vi "2D_Data_Interp.vi"() -> ()   [LabVIEW 2016]
uses:
  <vilib>/Math Plots/3D Math Plots/3D Surface/3D Surface XCtrl/3D Surface.xctl
  <vilib>/gmath/interp.llb/Interpolate 2D (2d X,Y).vi
  <vilib>/gmath/interp.llb/Create Mesh Grid (2D) (x,y arrays).vi
  <vilib>/Math Plots/3D Math Plots/3D Surface/3D Surface Datatype/Public/Plot Helper (Matrix).vi
  <vilib>/gmath/NI_Gmath.lvlib
  <vilib>/Math Plots/3D Math Plots/3D Surface/3D Surface Datatype/3D Surface Datatype.lvclass
  <vilib>/measure/NI_MABase.lvlib
  <vilib>/picture/3D Picture Control/NI_3D Picture Control.lvlib
panel:
  in  "Differential Conductance":dbl[][](graph)=[[172.002], [172.014], [172.02], [172.032], [172.05], [172.038], [171.99], [171.984], [172.008], [172.02], [172.038], [172.032], [172.008], [171.99], [171.984], [171.99], [172.008], [172.02], [172.032], [171.996], [172.002], [172.014], [172.032], [172.056], [172.056], [172.038], [172.008], [171.996], [172.014], [172.026], [172.032], [172.044], [172.008], [171.996], [171.99], [172.014], [172.032], [172.038], [172.032], [171.99], [171.984], [171.996], [172.014], [172.032], [172.026], [172.002], [171.99], [171.996], [172.02], [172.038], [172.05], [172.032], [172.002], [172.008], [172.014], [172.032], [172.044], [172.056], [172.044], [172.002], [171.996], [172.002], [172.026], [172.038], [172.044], [172.05], [172.02], [172.002], [171.99], [172.002], [172.008], [172.026], [172.02], [171.978], [171.978], [171.984], [171.99], [171.99], [172.002], [171.978], [171.96], [171.972], [171.984], [171.99], [171.996], [171.996], [171.978], [171.954], [171.948], [171.972], [171.99], [172.008], [172.032], [172.014], [171.996], [172.008], [172.014], [172.014], [172.008], [171.99], [171.972], [171.972], [171.99], [172.008], [172.032], [172.02], [171.996], [171.984], [171.996], [172.014], [172.02], [172.002], [171.972], [171.978], [171.99], [172.008], [172.026], [172.026], [171.99], [171.978], [171.99], [171.996], [172.002], [172.002], [172.002]]
  in  "ntimes":i32=5
  in  "sampling info 2":cluster{"Fs":dbl, "#s":dbl}={"Fs"=4.0, "#s"=2.0}
  out "Waveform Graph 2":waveform(dbl)(graph)
  in  "sampling info":cluster{"Fs":dbl, "#s":dbl}={"Fs"=4.0, "#s"=2.0}
  out "Waveform Graph":waveform(dbl)(graph)
  out "3D Surface":refnum<class "3D Plot Datatype.lvclass">[](xcontrol)
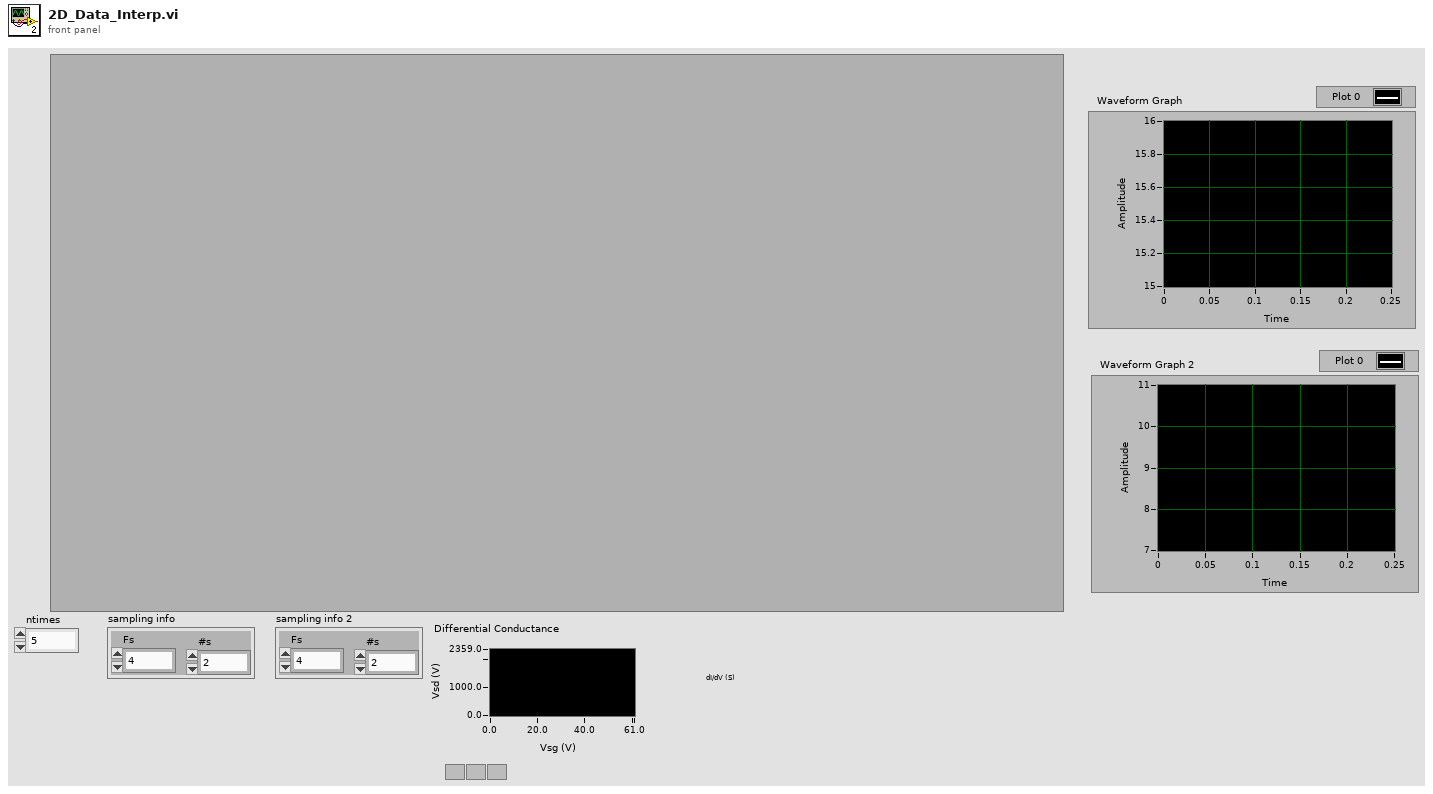
[diagram p1: front panel]
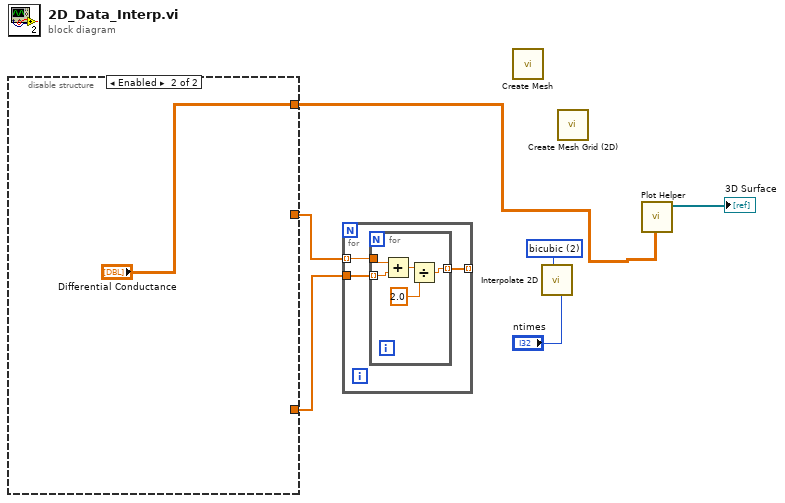
[diagram p0: block diagram]
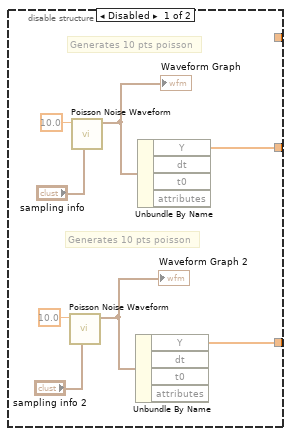
[diagram p2: hidden frame]
diagram:
  w3 = 2 items=["nearest", "bilinear", "bicubic", "bicubic spline"] ("method")
  n1 = disable-structure shown="Enabled" {
    disable-tunnel: [w8 _] -> w5
    disable-tunnel: [w7 _] -> w4
    disable-tunnel: [_ "Differential Conductance"] -> w1
    frame Disabled {
      # "Generates 10 pts poisson"
      # "Generates 10 pts poisson"
      n2 = call <vilib>:"Poisson Noise Waveform.vi"("sampling info"="sampling info 2", "mean"=10.0) -> ("signal out"=w10:waveform(dbl))  [unwired: 8 in, 1 out]
      "Waveform Graph 2" <- w10
      n3 = call <vilib>:"Poisson Noise Waveform.vi"("sampling info"="sampling info", "mean"=10.0) -> ("signal out"=w13:waveform(dbl))  [unwired: 8 in, 1 out]
      "Waveform Graph" <- w13
      n4 = Unbundle By Name(w10) -> ("Y"=w7:dbl[])  [unwired: 3 out]
      n5 = Unbundle By Name(w13) -> ("Y"=w8:dbl[])  [unwired: 3 out]
    }
    frame Enabled {
    }
  }
  n6 = for {
    tunnel: w5 -> [w18] mode=indexing
    tunnel: w4 -> [w17]
    tunnel: [w16] -> _ mode=indexing
    n7 = for {
      tunnel: w18 -> [w21]
      tunnel: w17 -> [w20] mode=indexing
      tunnel: [w23] -> w16 mode=indexing
      n8 = Add(x=w21, y=w20) -> (x+y=w22:dbl)
      n9 = Divide(x=w22, y=2.0) -> (x/y=w23:dbl)
    }
  }
  n10 = call <vilib>:"Create Mesh.vi"() -> ()  [unwired: 10 in, 2 out]
  n11 = call-poly <vilib>:"Interpolate 2D.vi"("ntimes"="ntimes", "method"=w3) -> ()  [unwired: 6 in, 4 out]
  n12 = call-poly <vilib>:"Create Mesh Grid (2D).vi"() -> ()  [unwired: 9 in, 3 out]
  n13 = call-poly <vilib>:"Plot Helper.vi"("z matrix"=w1) -> ("3D Plot lvclass Array out"=→"3D Surface":refnum<class "3D Plot Datatype.lvclass">[])  [unwired: 5 in, 5 out]
